vi "PassReceiverRole.vi"(6 "Tactic index in":i32, 7 "first call":bool, 8 "error in (no error)":errorcluster, 10 "Game in":refnum<class "Game.lvclass">, 11 "PassReceiverRole in":refnum<class "PassReceiverRole.lvclass">) -> (0 "error out":errorcluster, 1 "tactic index":i32, 2 "Robot out":refnum<class "Robot.lvclass">, 3 "PassReceiverRole out":refnum<class "PassReceiverRole.lvclass">)   [LabVIEW 2023, in "PassReceiverRole.lvclass"]
uses:
  PassReceiverRole.lvclass
  Robot_class/Robot.lvclass
  Game_class/Game.lvclass
  Utilities_class/Utilities.lvclass
  Role_class/Role.lvclass/Role.ctl
  PassReceiverRole.lvclass/PassReceiverRole.ctl
  Tacticbook_class/Tacticbook.lvclass/Tacticbook.ctl
  ShootTactic_class/States.ctl
  ShootTactic_class/ShootTactic.lvclass/ShootTactic.ctl
  Tacticbook_class/Read WaitPassTactic.vi
  Tacticbook_class/Write WaitPassTactic.vi
  Tacticbook_class/Read ShootTactic.vi
  ShootTactic_class/Read States.vi
  Tacticbook_class/Write ShootTactic.vi
  Role_class/Read Tacticbook.vi
  Read number_of_tactics.vi
  Role_class/Write Tacticbook.vi
  Role_class/Write tactic_index.vi
  Role_class/Read RobotRef.vi
  Tacticbook_class/Tacticbook.lvclass
  WaitPassTactic_class/WaitPassTactic.lvclass
  ShootTactic_class/ShootTactic.lvclass
panel:
  out "Game out":refnum<class "Game.lvclass">
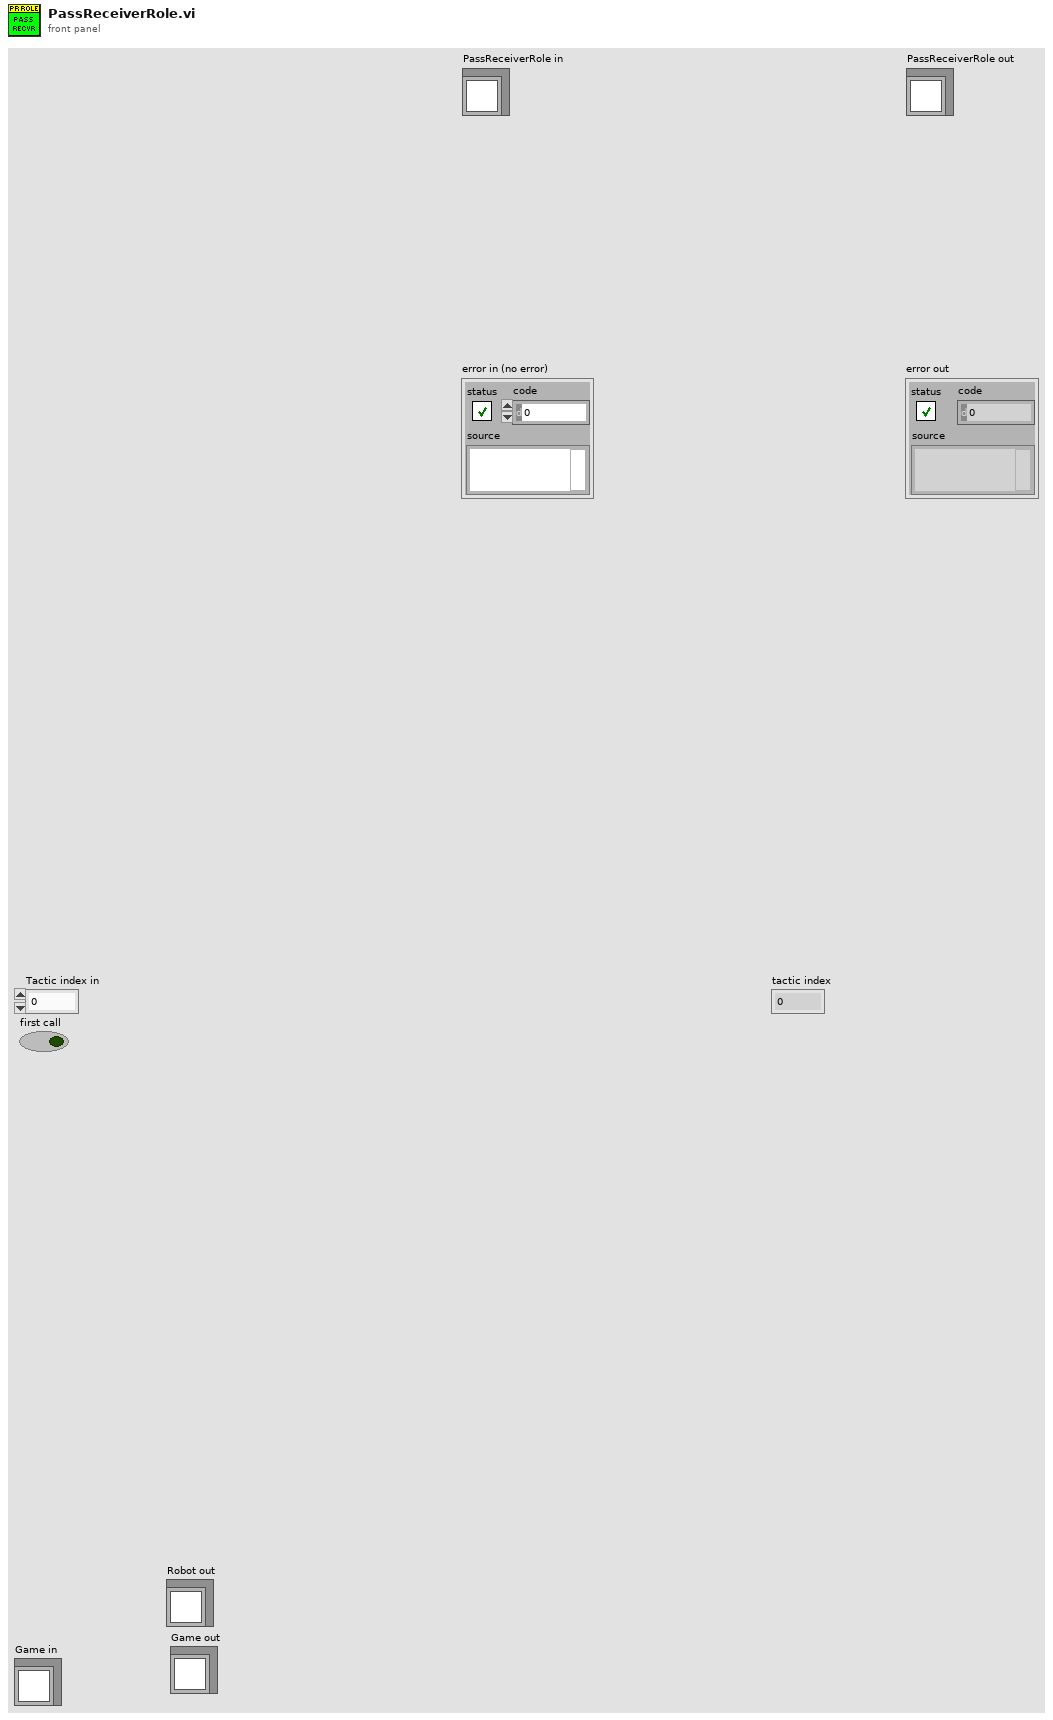
[diagram p1: front panel]
types:
  T1 = typedef "ShootTactic.lvclass/States.ctl" = enum16{"BallInGoalieArea", "Exit", "KickToGoal", "StealBall"}
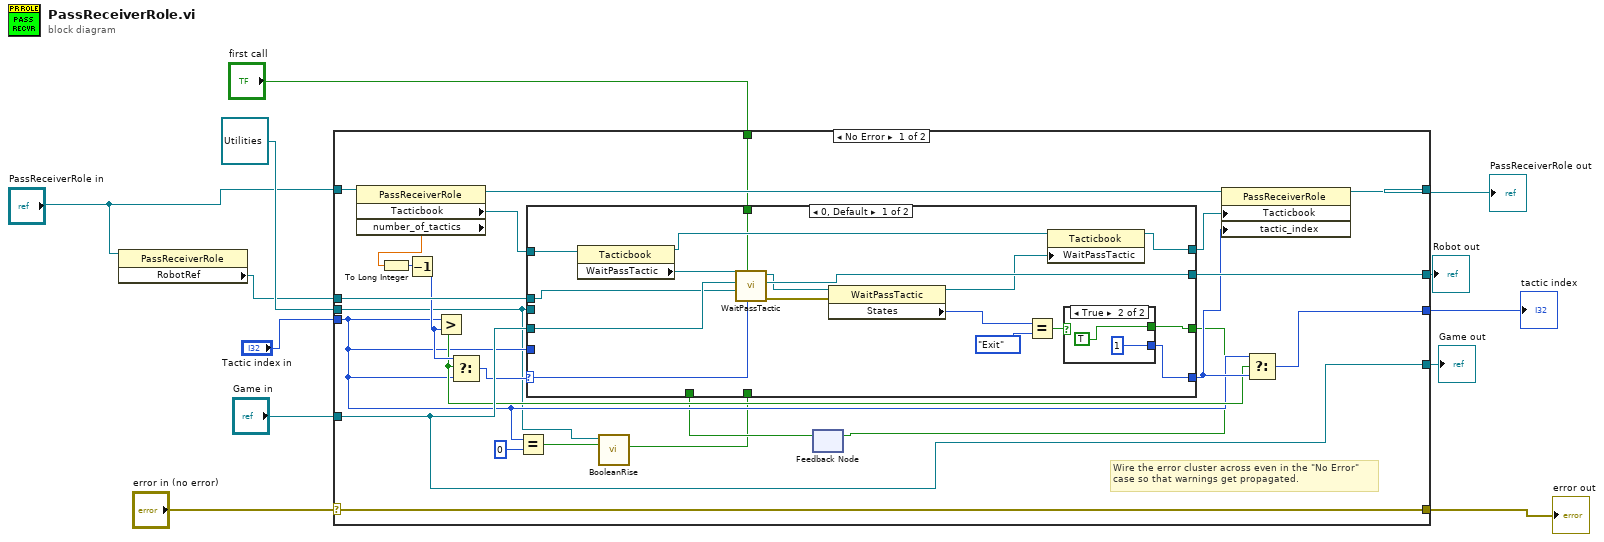
[diagram p0: block diagram]
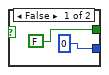
[diagram p2: hidden frame]
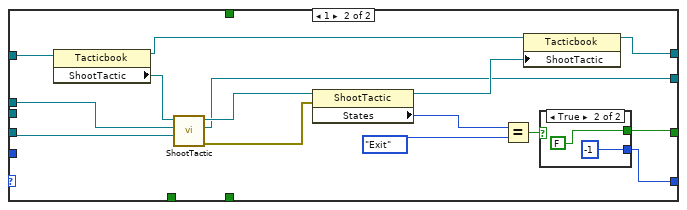
[diagram p3: hidden frame]
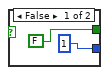
[diagram p4: hidden frame]
diagram:
  n1 = property class="PassReceiverRole"(reference="PassReceiverRole in") -> ("RobotRef"=w2:refnum<class "Robot.lvclass">)  [unwired: 1 in, 2 out]
  n2 = case shown="No Error" "error in (no error)" {
    selector: "error in (no error)" -> [w36 w80]
    tunnel: [w36 w80] -> w7
    tunnel: [w34 w79] -> w8
    tunnel: "PassReceiverRole in" -> [w35 w79]
    tunnel: w2 -> [w31 w78]
    tunnel: [w30 w78] -> w12
    tunnel: [w28 w77] -> w11
    tunnel: "Game in" -> [w28 w77]
    tunnel: [w23 _] -> w6
    tunnel: "Tactic index in" -> [w22 _]
    tunnel: refnum<class "Utilities.lvclass"> refnum ("Utilities in") -> [w21 _]
    tunnel: "first call" -> [w20 _]
    frame No Error {
      # "Wire the error cluster across even in the \"No Error\"\ncase so that warnings get propagated."
      n3 = property class="PassReceiverRole"(reference=w35) -> (reference out=w33:refnum<class "PassReceiverRole.lvclass">, "Tacticbook"=w32:refnum<class "Tacticbook.lvclass">, "number_of_tactics"=w13:dbl)  [unwired: 1 in, 1 out]
      n4 = To Long Integer(number=w13) -> (32bit integer=w14:i32)
      n5 = Decrement(x=w14) -> (x-1=w27:i32)
      n6 = Greater?(x=w22, y=w27) -> (0:w24:bool)
      n7 = Select(t=w27, s=w24, f=w22) -> (s? t:f=w26:i32)
      n8 = Equal?(x=w22, y=0) -> (x = y?=w17:bool)
      n9 = call "BooleanRise.vi"("Boolean in"=w17, "Utilities in"=w21) -> ("Boolean"=w15:bool)  [unwired: 7 in, 2 out]
      n10 = feedback #1() -> (w18:bool)  [unwired: 1 in]
      n11 = case shown="0, Default" w26 {
        selector: w26 -> [w37 _]
        tunnel: [w41 w59] -> w25
        tunnel: w32 -> [w53 w68]
        tunnel: w31 -> [w44 w63]
        tunnel: [w52 w65] -> w30
        tunnel: [w48 w64] -> w29
        tunnel: w28 -> [w45 w62]
        tunnel: w22 -> [_ _]
        tunnel: w21 -> [_ _]
        tunnel: w20 -> [w39 _]
        tunnel: [w40 w60] -> w19
        tunnel: w18 -> [_ _]
        tunnel: w15 -> [_ _]
        frame 0, Default {
          n12 = property class="Tacticbook"(reference=w53) -> (reference out=w50:refnum<class "Tacticbook.lvclass">, "WaitPassTactic"=w47:refnum<class "WaitPassTactic.lvclass">)  [unwired: 1 in, 1 out]
          n13 = call-dynamic "WaitPassTactic.vi"("Tactic index in"=w37, "first call"=w39, "Robot"=w44, "Game in"=w45, "WaitPassTactic in"=w47) -> ("error out"=w51:errorcluster, "Robot out"=w52:refnum<class "Robot.lvclass">, "WaitPassTactic out"=w46:refnum<class "WaitPassTactic.lvclass">)  [unwired: 4 in]
          n14 = property class="WaitPassTactic"(reference=w46, error in=w51) -> (reference out=w49:refnum<class "WaitPassTactic.lvclass">, "States"=w42:enum16{"State 0", "State 1", "State 2", "Exit"})  [unwired: 1 out]
          n15 = Equal?(x=w42, y=enum16{"State 0", "State 1", "State 2", "Exit"}."Exit") -> (x = y?=w43:bool)
          n16 = property class="Tacticbook"(reference=w50, "WaitPassTactic"=w49) -> (reference out=w48:refnum<class "Tacticbook.lvclass">)  [unwired: 1 in, 1 out]
          n17 = case shown="True" w43 {
            tunnel: [0 1] -> w41
            tunnel: [FALSE TRUE] -> w40
            frame False {
            }
            frame True {
            }
          }
        }
        frame 1 {
          n18 = property class="Tacticbook"(reference=w68) -> (reference out=w72:refnum<class "Tacticbook.lvclass">, "ShootTactic"=w67:refnum<class "ShootTactic.lvclass">)  [unwired: 1 in, 1 out]
          n19 = call "ShootTactic.vi"("Game in"=w62, "Robot"=w63, "ShootTactic in"=w67) -> ("error out"=w61:errorcluster, "Robot out"=w65:refnum<class "Robot.lvclass">, "ShootTactic out"=w66:refnum<class "ShootTactic.lvclass">)  [unwired: 6 in]
          n20 = property class="ShootTactic"(reference=w66, error in=w61) -> (reference out=w71:refnum<class "ShootTactic.lvclass">, "States"=w69:T1)  [unwired: 1 out]
          n21 = Equal?(x=w69, y=States."Exit" ("States")) -> (x = y?=w70:bool)
          n22 = property class="Tacticbook"(reference=w72, "ShootTactic"=w71) -> (reference out=w64:refnum<class "Tacticbook.lvclass">)  [unwired: 1 in, 1 out]
          n23 = case shown="True" w70 {
            tunnel: [1 -1] -> w59
            tunnel: [FALSE FALSE] -> w60
            frame False {
            }
            frame True {
            }
          }
        }
      }
      n24 = feedback-in #1(w19) -> ()
      n25 = property class="PassReceiverRole"(reference=w33, "Tacticbook"=w29, "tactic_index"=w25) -> (reference out=w34:refnum<class "PassReceiverRole.lvclass">)  [unwired: 1 in, 1 out]
      n26 = Select(t=w22, s=w24, f=w25) -> (s? t:f=w23:i32)
    }
    frame Error {
    }
  }
  "error out" <- w7
  "PassReceiverRole out" <- w8
  "Robot out" <- w12
  "Game out" <- w11
  "tactic index" <- w6
